vi "Analyse.vi"(8 "error in (no error)":errorcluster, 10 "ImageData":T1, 11 "ImageAnalyser in":refnum<class "ImageAnalyser.lvclass">) -> (0 "error out":errorcluster, 3 "ImageAnalyser out":refnum<class "ImageAnalyser.lvclass">)   [LabVIEW 2011, in "Tools.lvlib" / "Imaging.lvlib" / "ImageAnalyser.lvclass"]
uses:
  ImageAnalyser.lvclass
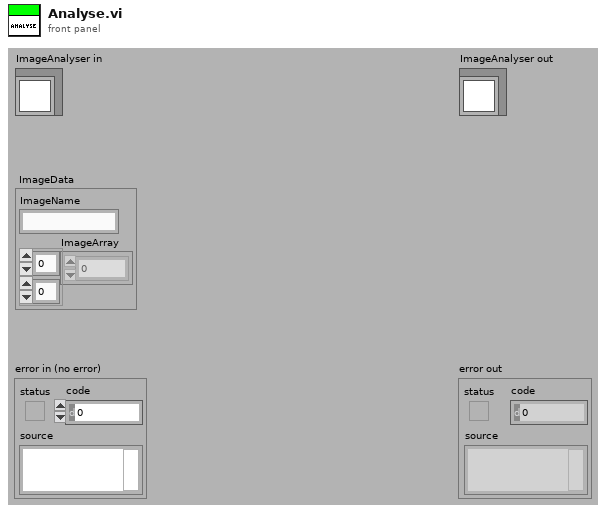
[diagram p1: front panel]
types:
  T1 = cluster{"ImageName":string, "ImageArray":sgl[][]}
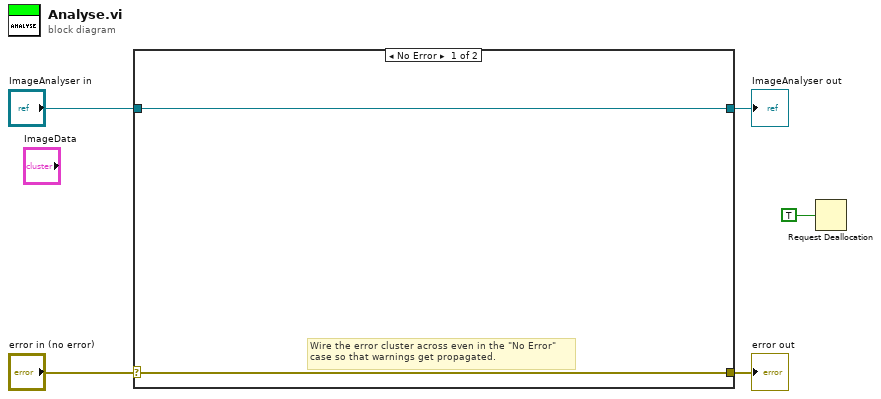
[diagram p0: block diagram]
diagram:
  n1 = case shown="No Error" "error in (no error)" {
    selector: "error in (no error)" -> [w6 w9]
    tunnel: [w6 w9] -> w4
    tunnel: [w7 w8] -> w2
    tunnel: "ImageAnalyser in" -> [w7 w8]
    frame No Error {
      # "Wire the error cluster across even in the \"No Error\"\ncase so that warnings get propagated."
    }
    frame Error {
    }
  }
  "error out" <- w4
  "ImageAnalyser out" <- w2
  n2 = Request Deallocation(TRUE ("flag")) -> ()
